vi "Calc Currente Exposure Time.vi"(8 "error in (no error)":errorcluster, 11 "CCDCamera in":refnum<class "Simulated Camera.lvclass">) -> (0 "error out":errorcluster, 3 "CCDCamera out":refnum<class "Simulated Camera.lvclass">)   [LabVIEW 2018, in "Simulated Camera.lvclass"]
doc: "Calculate the exposure time of the current acquisition\n\nThis calculation is based on the timestamp get after the star of the acquisition"
uses:
  Simulated Camera.lvclass
  Simulated Camera.lvclass/Simulated Camera.ctl
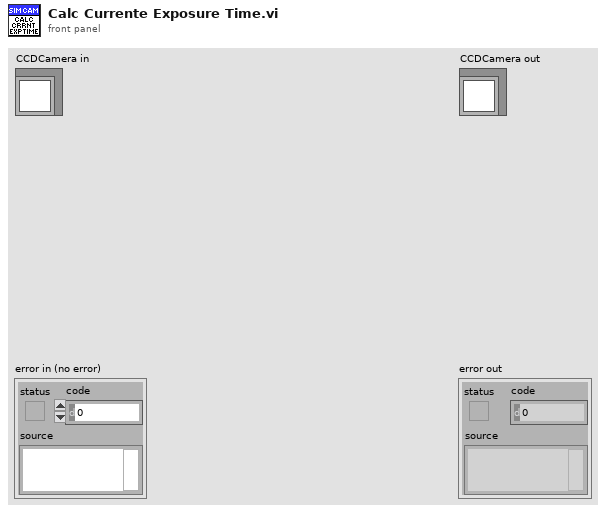
[diagram p1: front panel]
types:
  T1 = cluster{"CYCLES_DONE":u16, "LAST_IMAGE_NAME":string, "USED_DISK_SPACE":u16, "FRAMES_DONE":u16, "CCD_STATUS":string, "CURRENT_TEMPERATURE":i16, "TEMPERATURE_STATUS":string, "FRAME_EXPOSURE_TIME":sgl, "ERROR":bool, "SERIAL_NUMBER":u16, "ACQUIRING":bool, "IMAGE_INDEX":u32, "SEQS_DONE":u16}
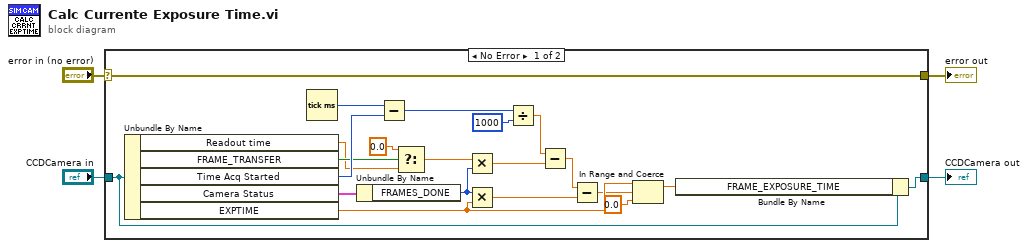
[diagram p0: block diagram]
diagram:
  n1 = case shown="No Error" "error in (no error)" {
    selector: "error in (no error)" -> [w7 w27]
    tunnel: [w7 w27] -> w2
    tunnel: [w25 w26] -> w1
    tunnel: "CCDCamera in" -> [w13 w26]
    frame No Error {
      n2 = Unbundle By Name(w13) -> ("Readout time"=w6:dbl, "FRAME_TRANSFER"=w14:bool, "Time Acq Started"=w23:u32, "Camera Status"=w20:T1, "EXPTIME"=w19:dbl)
      n3 = Tick Count (ms)() -> (millisecond timer value=w24:u32)
      n4 = Unbundle By Name(w20) -> ("FRAMES_DONE"=w8:u16)
      n5 = Subtract(x=w24, y=w23) -> (x-y=w22:u32)
      n6 = Select(t=sgl 0.0, s=w14, f=w6) -> (s? t:f=w10:dbl)
      n7 = Multiply(x=w10, y=w8) -> (x*y=w9:dbl)
      n8 = Multiply(x=w8, y=w19) -> (x*y=w17:dbl)
      n9 = Divide(x=w22, y=1000) -> (x/y=w12:dbl)
      n10 = Subtract(x=w12, y=w9) -> (x-y=w11:dbl)
      n11 = Subtract(x=w11, y=w17) -> (x-y=w16:dbl)
      n12 = In Range and Coerce(upper limit=w19, x=w16, lower limit=sgl 0.0) -> (coerced(x)=w5:dbl)  [unwired: 1 out]
      n13 = Bundle By Name(cluster=w13, "FRAME_EXPOSURE_TIME"=w5) -> (w25:refnum<class "Simulated Camera.lvclass">)
    }
    frame Error {
    }
  }
  "error out" <- w2
  "CCDCamera out" <- w1
